vi "Lidar V3.1 RT Main.vi"() -> ()   [LabVIEW 2013]
uses:
  <vilib>/Platform/TimedLoop/XDataNode/timing_clust.ctl
  <vilib>/Platform/TimedLoop/XDataNode/nitl_modes.ctl
  <vilib>/Platform/TimedLoop/XDataNode/wakeup.ctl
  <vilib>/FPGAPlugInAG/PXIe-7962R/niLvFpga_Open_PXIe-7962R.vi
  <vilib>/rvi/interface/common/dynamic/niFpgaDynamicAddResources.vi
  <vilib>/FPGAPlugInAG/Dynamic/niLvFpga_Abort_Dynamic.vi
  <vilib>/FPGAPlugInAG/Dynamic/niLvFpga_Reset_Dynamic.vi
  <vilib>/rvi/interface/common/niFpgaWaitOnOcc.vi
  <vilib>/Utility/error.llb/Error Cluster From Error Code.vi
  <vilib>/FPGAPlugInAG/Dynamic/niLvFpga_Run_Dynamic.vi
  <vilib>/rvi/errors/niLvFpgaAdjustHostInterfaceError.vi
  <vilib>/FPGAPlugInAG/Dynamic/niLvFpga_Close_Dynamic.vi
  <vilib>/rvi/interface/nirviOpenFPGA/nirviOpenFPGA.xnode
  FPGA Bitfiles/GMLIDARV4_FPGATarget3_LIDARV3.1FPGAMai_NnL+G1AkDV4.lvbitx
  <vilib>/rvi/interface/nirviMethod/nirviMethod.xnode
  <vilib>/Platform/TimedLoop/XDataNode/XDataNode.xnode
  <vilib>/rvi/interface/nirviReadWriteControl/nirviReadWriteControl.xnode
  <vilib>/rvi/interface/nirviCloseFPGA/nirviCloseFPGA.xnode
  <vilib>/FPGAPlugInAG/Dynamic/niLvFpga_ReadFifo_Dynamic.vi
  <vilib>/rvi/errors/niLvFpgaMergeErrorWithErrorCode.vi
  <vilib>/ptbypt/NI_PtbyPt.lvlib
  NiFpgaLv.dll
  <vilib>/rvi/interface/Simulation/niFpgaSimulationCallBeginRW.vi
  <vilib>/Platform/TimedLoop/XDataNode/XDNodeRunTimeDep.lvlib
  <vilib>/FPGAPlugInAG/Dynamic/niLvFpga_StopFifo_Dynamic.vi
  <vilib>/FPGAPlugInAG/Dynamic/niLvFpga_ConfigureFifo_Dynamic.vi
  <vilib>/FPGAPlugInAG/Dynamic/niLvFpga_AcquireReadRegionFifo_Dynamic.vi
panel:
  in  "SubstractDark":bool
  out "file path mem":path=path "C:/Users/LIDAR/Desktop/Scans/Debug1.dat"
  in  "SaveDarkFile":bool
  out "Dark Data":dbl[](graph)
  in  "Fill Dark":bool
  in  "SampPerPulse":u16=100 caption="Samples Per Pulse"
  out "Actual Depth 2":u32=4000768
  in  "Mean":bool
  in  "Pilse Wait During Stream":u16=40
  out "SampMem":bool
  in  "# of Frames":u32=1 caption="# of Frames:"
  in  "Frames2File":bool
  in  "Fill VGA":bool
  in  "VGA data":i16[](array[numeric])=[0, 300, 600, 900, 1200, 1500, 1800, 2100, 2400, 2700, 3000, 3300, 3600, 3900, 4200, 4500, 4800, 5100, 5400, 5700, 6000, 6300, 6600, 6900, 7200, 7500, 7800, 8100, 8400, 8700, 9000, 9300, 9600, 9900, 10200, 10500, 10800, 11100, 11400, 11700, 12000, 12300, 12600, 12900, 13200, 13500, 13800, 14100, 14400, 14700, 15000, 15300, 15600, 15900, 16200, 16500, 16800, 17100, 17400, 17700, 18000, 18300, 18600, 18900, 19200, 19500, 19800, 20100, 20400, 20700, 21000, 21300, 21600, 21900, 22200, 22500, 22800, 23100, 23400, 23700, 24000, 24300, 24600, 24900, 25200, 25500, 25800, 26100, 26400, 26700, 27000, 27300, 27600, 27900, 28200, 28500, 28800, 29100, 29400, 29700]
  in  "PulsePerLed":i16=200 caption="Pulses Per Led"
  in  "ScanMode":bool
  in  "FrameStartDisable":bool=TRUE
  out "# of Frames 2":u32
  in  "Frames Stream":bool
  in  "Frames Period":i64=100
  out "Mean Data Timeouts":u16=31333
  out "Actual Depth":u32=4000768
  out "Raw Data Timeouts":u16
  in  "StreamToRawFile":bool
  in  "SingleFrame":bool
  in  "SamplingEnable":bool
  out "Elements":i32=8192
  out "DiskWritesCounter":dbl=6240.0
  out "error out":errorcluster
  in  "Write To File":bool
  in  "file path (use dialog)":path=path "C:/Users/LIDAR/Desktop/Scans/Debug1.dat"
  out "Elements Remaining":u32
  in  "MaxStartSample":u8
  out "Intensity Map":i32[][](graph)=[[4194249, 188752, 224556, 243564, 289464, 295370, 311361, 314977, 331462, 330943, 315425, 258027, 251933, 242647, 177250, 117913], [200096, 226594, 258129, 270777, 343444, 323211, 332534, 349964, 357344, 353930, 351094, 316150, 294820, 265633, 227733, 171654], [232886, 270088, 321175, 342251, 368583, 361813, 383924, 347348, 410423, 416541, 367914, 380971, 350571, 312824, 273514, 214192], [239958, 294260, 316500, 326793, 374683, 379303, 387592, 379517, 393877, 417364, 396781, 427517, 386177, 339906, 293385, 246523], [260822, 288128, 359883, 369758, 370777, 382402, 409421, 424013, 426403, 411324, 377639, 397431, 416573, 383670, 322005, 280464], [293823, 329912, 354981, 353022, 396436, 401968, 405276, 416671, 420226, 421228, 384422, 394623, 423961, 381848, 346743, 317362], [310692, 338310, 379615, 380848, 383413, 440416, 444786, 422715, 400342, 437502, 444652, 443019, 440346, 454579, 408555, 369326], [316804, 342015, 359690, 380257, 428896, 414631, 434872, 421060, 458914, 427260, 480766, 417432, 468249, 416307, 402490, 365401], [303901, 338915, 339851, 378333, 398332, 440528, 418068, 439806, 390220, 406181, 407082, 381751, 436716, 400796, 381358, 367759], [295709, 371852, 371391, 347317, 360777, 398739, 412251, 396109, 380118, 408733, 405717, 414557, 407467, 386729, 398829, 360545], [314919, 350825, 374405, 365676, 393860, 415850, 410229, 441555, 421003, 421694, 496428, 416662, 416732, 423847, 410450, 407682], [328113, 313254, 370853, 381700, 393710, 410688, 382753, 449829, 443229, 458715, 431022, 404412, 413198, 434281, 400200, 423687], [304084, 349902, 347341, 353314, 401704, 422113, 414195, 423142, 395933, 398360, 432970, 390996, 385527, 379727, 377788, 346075], [283824, 313637, 343405, 347712, 394807, 379854, 411027, 383672, 370711, 368886, 401373, 375390, 385415, 371526, 399492, 384905], [260891, 301413, 328721, 319057, 369689, 372537, 399083, 380860, 364897, 382376, 427845, 447504, 378799, 362669, 372146, 366827], [260673, 275664, 297429, 325884, 386054, 389853, 378447, 387074, 385946, 363162, 422310, 380432, 373896, 375205, 367301, 363228], [275808, 284523, 294765, 333943, 308894, 378299, 378336, 357836, 389531, 381008, 372799, 357010, 370219, 350399, 328994, 324885], [232169, 242832, 279229, 299502, 307673, 352062, 346701, 334907, 340086, 344861, 384207, 371964, 357009, 350037, 361186, 312514], [217595, 247026, 267875, 295673, 319858, 333157, 327430, 316329, 320075, 324786, 310662, 357832, 315871, 368283, 331984, 254258], [210648, 254981, 278468, 289551, 280066, 318278, 342140, 319921, 320714, 335552, 365830, 364916, 332478, 350151, 315016, 244036]]
  in  "ActiveLedIndex":u16=144
  in  "LedScanDebEn":bool
  in  "LaserPower 1":bool=TRUE
  in  "LaserPower 0":bool=TRUE
  out "Range Map":u32[][](graph)=[[0, 62009, 61985, 61985, 62033, 61985, 61985, 62033, 62033, 62033, 62057, 62165, 62117, 62033, 62117, 62357], [61865, 61925, 62021, 61985, 62057, 62045, 62081, 62129, 62093, 62093, 62069, 62057, 62069, 62069, 62021, 61985], [62201, 62285, 62261, 62321, 62297, 62357, 62357, 62393, 62189, 62213, 62225, 62189, 62201, 62261, 62321, 62357], [62381, 62357, 62405, 62357, 62333, 62381, 62393, 62429, 62297, 62297, 62285, 62297, 62285, 62273, 62297, 62357], [61841, 61901, 61997, 61973, 61973, 62045, 62009, 62033, 62081, 62081, 62117, 62069, 62105, 61997, 62033, 61961], [61973, 61961, 61973, 61961, 61997, 62033, 62033, 62057, 62117, 62081, 62141, 62141, 62117, 62069, 62009, 61973], [62201, 62249, 62237, 62249, 62285, 62285, 62249, 62297, 62201, 62189, 62177, 62225, 62177, 62117, 62069, 62105], [62261, 62357, 62357, 62357, 62297, 62381, 62357, 62357, 62189, 62273, 62225, 62297, 62261, 62273, 62201, 62141], [61709, 61745, 61757, 61733, 61733, 61745, 61769, 61793, 61889, 61901, 61901, 61937, 61913, 61889, 61877, 61841], [61721, 61733, 61745, 61733, 61745, 61757, 61745, 61781, 61901, 61877, 61913, 61925, 61937, 61865, 61865, 61841], [62009, 62009, 62033, 62021, 61997, 62009, 62021, 62021, 61949, 61973, 61949, 61997, 62009, 61961, 61973, 61937], [61853, 61889, 61889, 61853, 61877, 61877, 61901, 61865, 61757, 61793, 61805, 61841, 61841, 61793, 61793, 61781], [61541, 61541, 61565, 61541, 61541, 61541, 61541, 61565, 61589, 61613, 61625, 61637, 61637, 61601, 61613, 61625], [61733, 61733, 61733, 61721, 61721, 61733, 61733, 61721, 61781, 61793, 61829, 61817, 61829, 61817, 61817, 61829], [61769, 61769, 61769, 61769, 61745, 61769, 61793, 61781, 61709, 61721, 61697, 61733, 61733, 61733, 61709, 61709], [61769, 61781, 61805, 61769, 61745, 61781, 61793, 61793, 61673, 61721, 61709, 61709, 61721, 61697, 61709, 61685], [61541, 61541, 61541, 61517, 61529, 61565, 61565, 61529, 61577, 61577, 61589, 61589, 61601, 61565, 61577, 61589], [61529, 61505, 61529, 61505, 61541, 61529, 61529, 61529, 61589, 61589, 61637, 61625, 61637, 61613, 61625, 61601], [61745, 61745, 61745, 61733, 61721, 61733, 61745, 61745, 61673, 61685, 61685, 61697, 61709, 61685, 61673, 61721], [61637, 61601, 61625, 61601, 61613, 61625, 61625, 61625, 61553, 61553, 61553, 61577, 61589, 61553, 61553, 31574]]
  in  "PulseEndClock":u8=4
  in  "PulseWaitClck":u16
  in  "Freq [Mhz]":dbl=125000000.0 format="%#_6p"
  out "standard deviation":dbl format="%0.5f"
  out "Distance":dbl format="%#.4f"
  in  "stop":bool=TRUE
  # "Auto Actions"
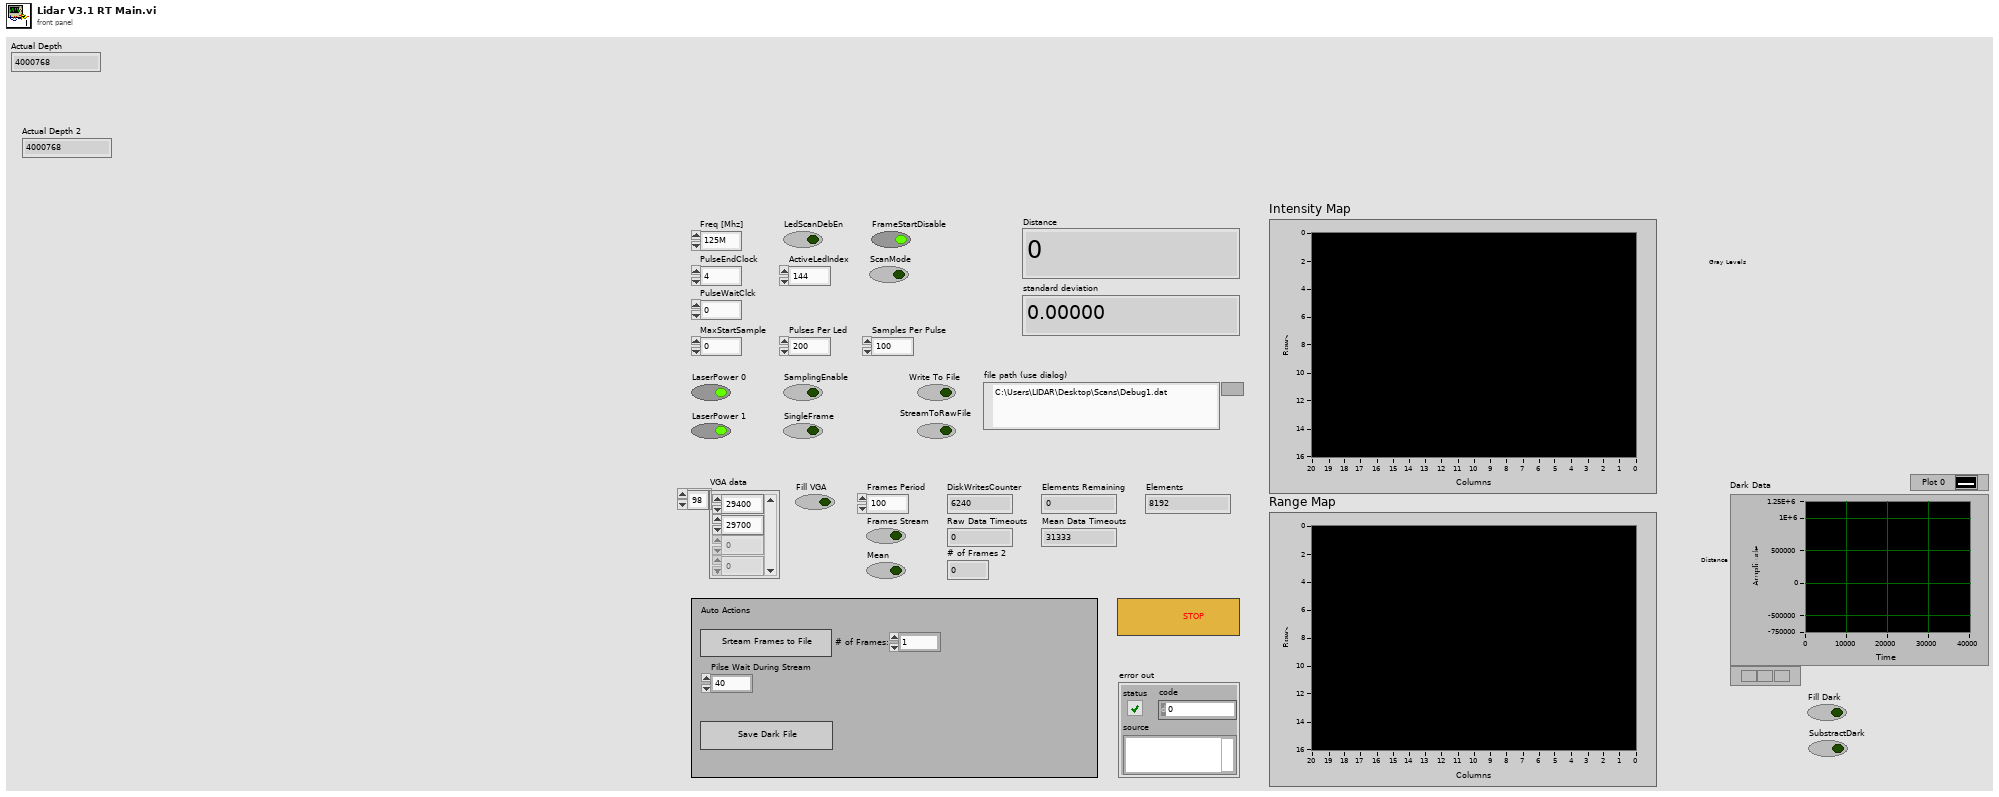
[diagram p1: front panel]
types:
  T1 = typedef "XDNodeRunTimeDep.lvlib/timing_clust.ctl" = cluster{"Expected End [f-1]":u64, "Actual End [f-1]":u64, "Finished Late? [f-1]":bool, "Expected End [i-1]":u64, "Actual End [i-1]":u64, "Finished Late? [i-1]":bool, "Expected Start [i]":u64, "Actual Start [i]":u64, "Expected Start [f]":u64, "Actual Start [f]":u64, "Source Name":string, "Structure Name":string, "Period":i64, "Deadline":i64, "Offset":i64, "Start":i64, "Priority":i32, "Timeout":i32, "Mode":T2, "Wakeup Reason":T3, "Error":errorcluster, "Source Type":string, "Secondary Source Type":string, "Global End Time":u64, "Global Start Time":u64, "Frame Duration":u64, "Iteration Duration":u64, "Assigned CPU":i32, "I/O Scan Engine Mode":u32}
  T2 = typedef "XDNodeRunTimeDep.lvlib/nitl_modes.ctl" = enum32{"No Change", "Process missed periods, maintain original phase", "Discard missed periods, maintain original phase", "Process missed periods, ignore original phase", "Discard missed periods, ignore original phase"}
  T3 = typedef "XDNodeRunTimeDep.lvlib/wakeup.ctl" = enum32{"Normal", "Aborted", "Asynchronous wakeup", "Timing source error", "Timed loop error", "Timeout"}
  T4 = enum16{"open", "replace", "create", "open or create", "replace or create", "replace or create with confirmation"}
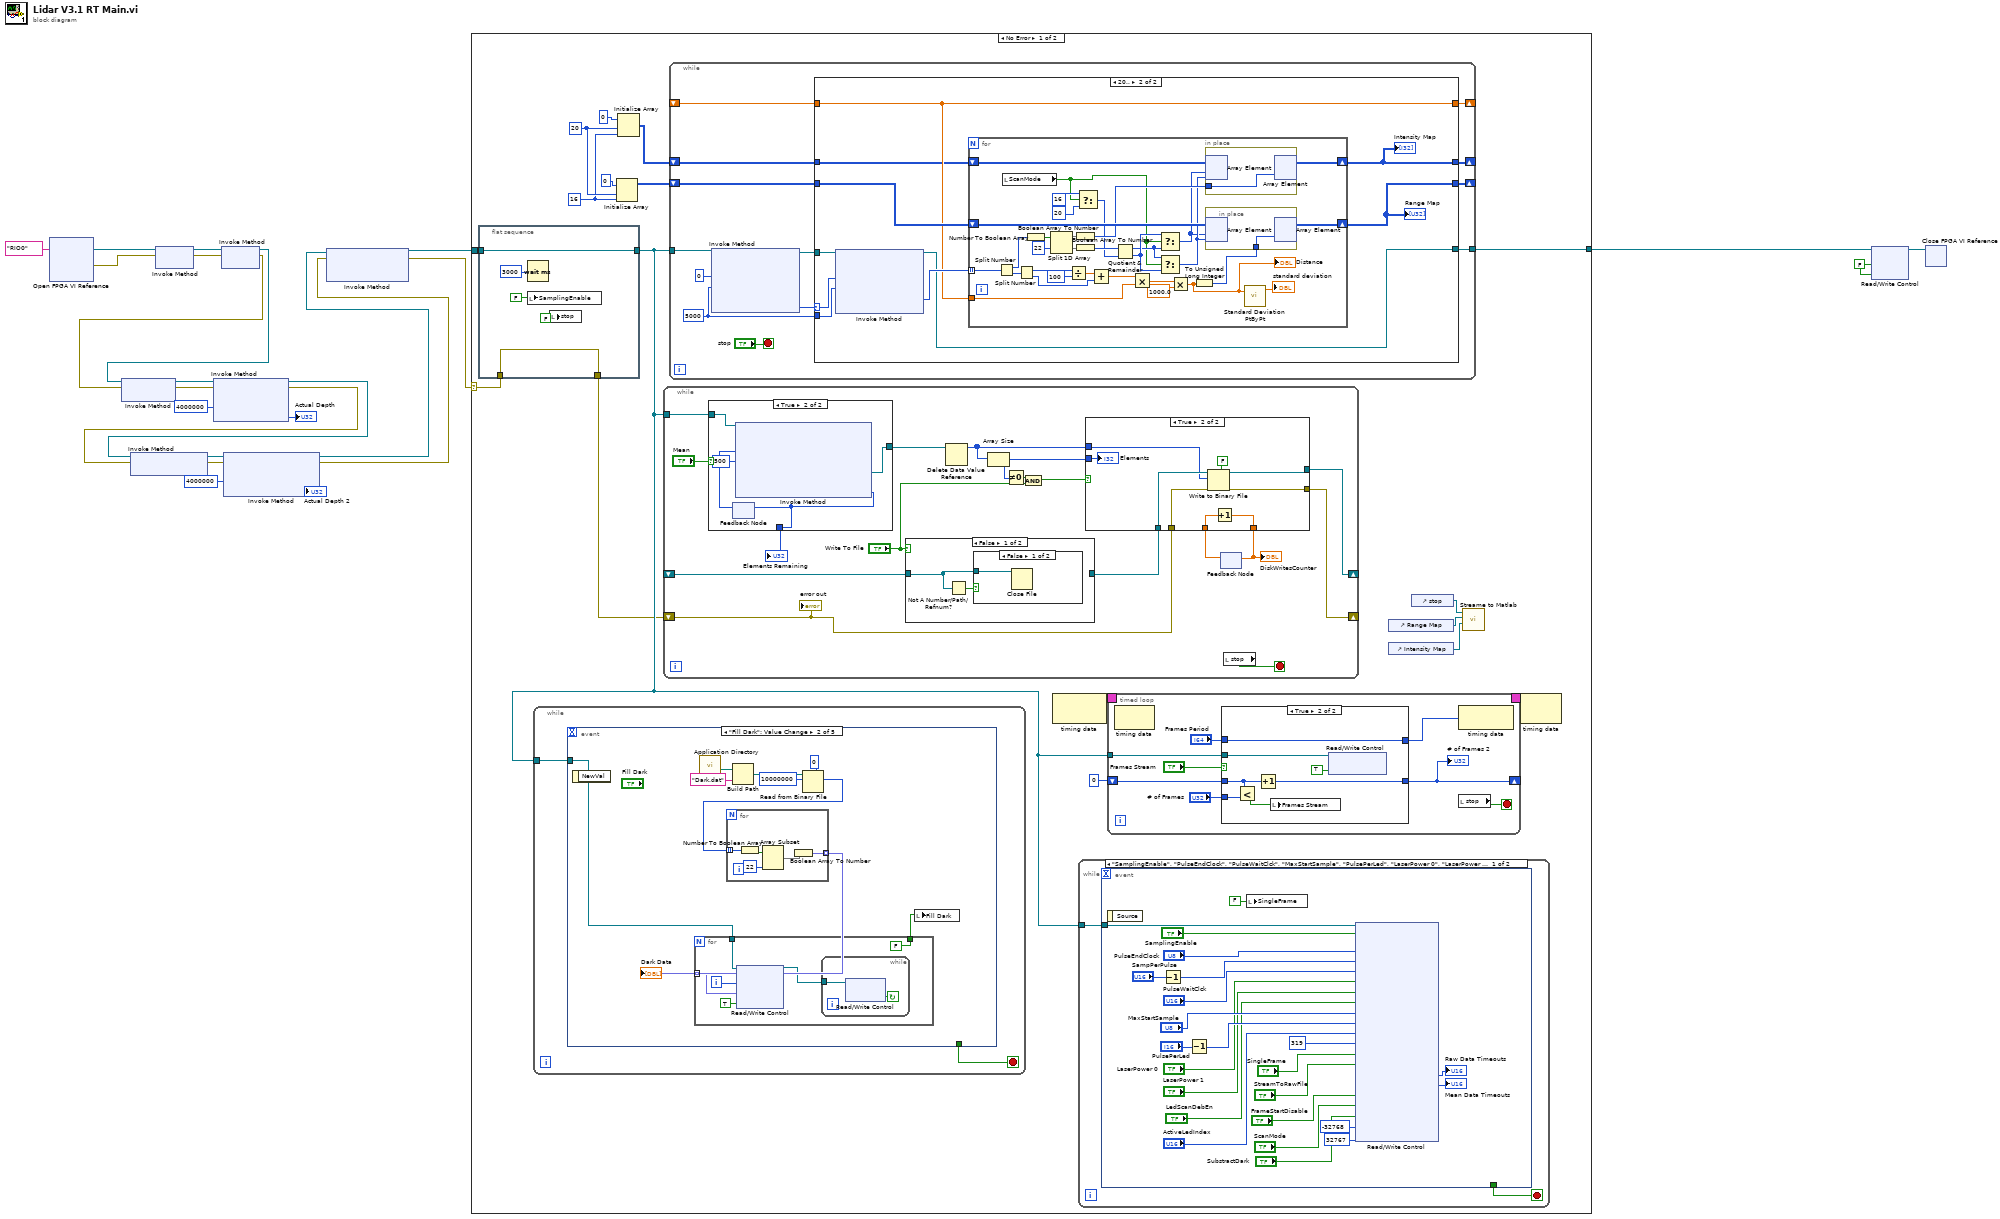
[diagram p0: block diagram]
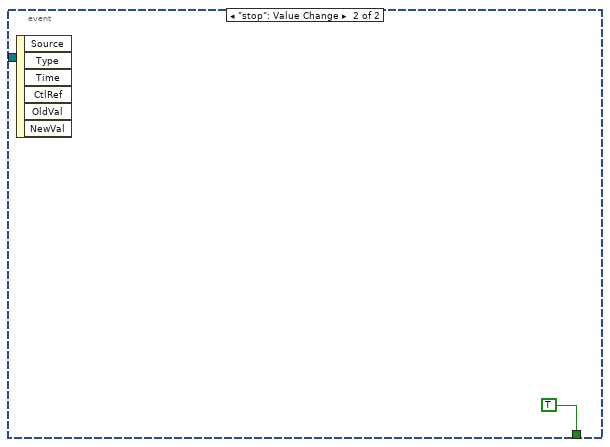
[diagram p2: hidden frame]
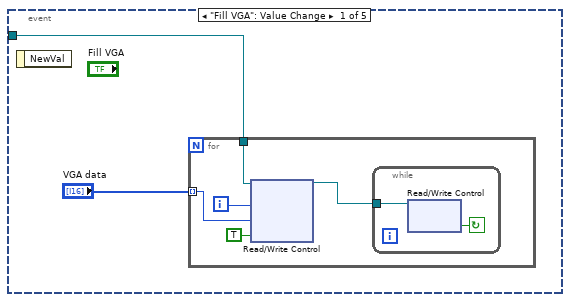
[diagram p3: hidden frame]
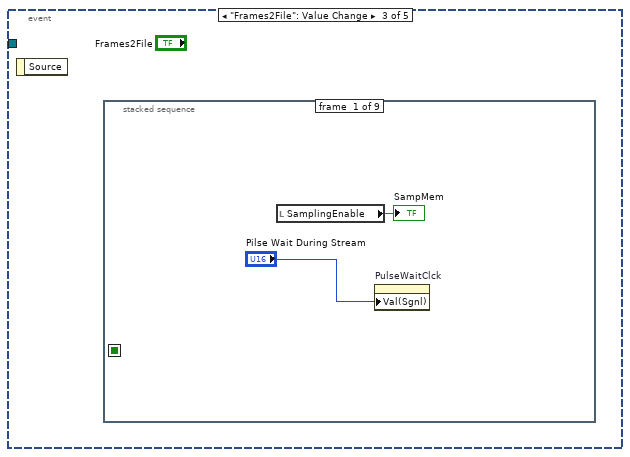
[diagram p4: hidden frame]
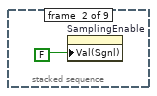
[diagram p5: hidden frame]
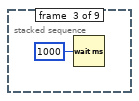
[diagram p6: hidden frame]
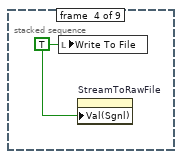
[diagram p7: hidden frame]
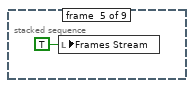
[diagram p8: hidden frame]
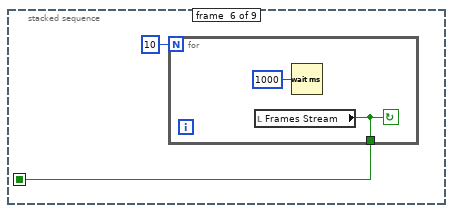
[diagram p9: hidden frame]
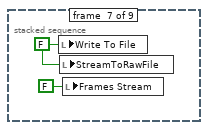
[diagram p10: hidden frame]
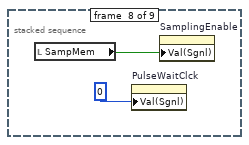
[diagram p11: hidden frame]
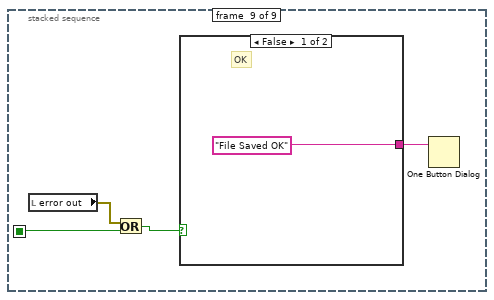
[diagram p12: hidden frame]
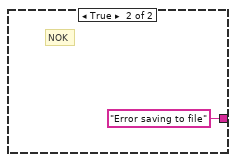
[diagram p13: hidden frame]
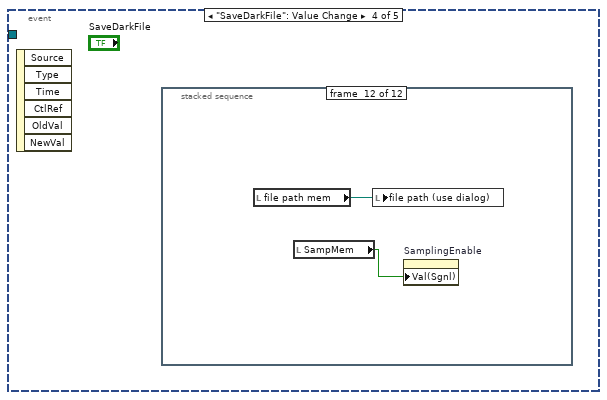
[diagram p14: hidden frame]
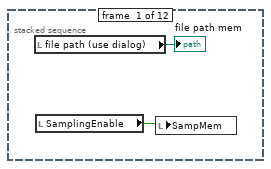
[diagram p15: hidden frame]
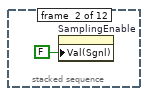
[diagram p16: hidden frame]
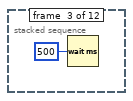
[diagram p17: hidden frame]
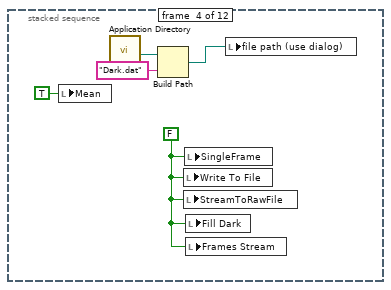
[diagram p18: hidden frame]
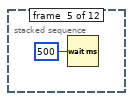
[diagram p19: hidden frame]
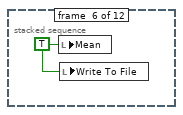
[diagram p20: hidden frame]
diagram:
  w14 = FALSE ("PFI2")
  n1 = xnode "Open FPGA VI Reference"("resource name"=tag "RIO0") -> ("FPGA VI Reference Out"=w22:refnum<k20>, "error out"=w20:errorcluster)  [unwired: 1 in]
  n2 = xnode "Invoke Method"("FPGA VI Reference In"=w22, "error in"=w20) -> ("FPGA VI Reference Out"=w21:refnum<k20>, "error out"=w19:errorcluster)
  n3 = xnode "Invoke Method"("FPGA VI Reference In"=w21, "error in"=w19) -> ("FPGA VI Reference Out"=w6:refnum<k20>, "error out"=w5:errorcluster)
  n4 = xnode "Invoke Method"("FPGA VI Reference In"=w6, "error in"=w5) -> ("FPGA VI Reference Out"=w17:refnum<k20>, "error out"=w18:errorcluster)
  n5 = xnode "Invoke Method"("FPGA VI Reference In"=w17, "error in"=w18, "Requested Depth"=u32 4000000) -> ("FPGA VI Reference Out"=w8:refnum<k20>, "error out"=w7:errorcluster, "Actual Depth"=→"Actual Depth":u32)
  n6 = xnode "Invoke Method"("FPGA VI Reference In"=w8, "error in"=w7) -> ("FPGA VI Reference Out"=w10:refnum<k20>, "error out"=w9:errorcluster)
  n7 = xnode "Invoke Method"("FPGA VI Reference In"=w10, "error in"=w9, "Requested Depth"=u32 4000000) -> ("FPGA VI Reference Out"=w4:refnum<k20>, "error out"=w2:errorcluster, "Actual Depth"=→"Actual Depth 2":u32)
  n8 = xnode "Invoke Method"("FPGA VI Reference In"=w4, "error in"=w2) -> ("FPGA VI Reference Out"=w3:refnum<k20>, "error out"=w1:errorcluster)  [unwired: 1 in]
  n9 = case shown="No Error" w1 {
    selector: w1 -> [w29 w285]
    tunnel: [w39 w286] -> w23
    tunnel: w3 -> [w31 w286]
    frame No Error {
      w32 = 16 ("dimension size")
      w36 = 20 ("dimension size")
      n10 = flat-sequence {
        tunnel: [w145] -> w30
        tunnel: w31 -> [w145]
        tunnel: w29 -> [w141]
        tunnel: [w141] -> w28
        frame #0 {
          n11 = Wait (ms)(milliseconds to wait=u32 3000) -> ()  [unwired: 1 out]
          n12 = local write "SamplingEnable"(FALSE ("SamplingEnable")) -> ()
          n13 = local write "stop"(FALSE ("stop")) -> ()
        }
      }
      n14 = while {
        tunnel: w30 -> [w70]
        stop <- w69 stop-if-true
        n15 = event shown="[1] \"Fill Dark\": Value Change" {
          selector: _ -> [_ _ _ _ _]
          dyn-events: _ -> [_ _ _ _ _]
          timeout: _ -> [_ _ _ _ _]
          tunnel: w70 -> [w71 w83 _ _ _]
          tunnel: [_ _ _ _ TRUE] -> w69
          event "Fill VGA": Value Change {
            n16 = event-data() -> ()  [unwired: 1 in, 1 out]
            n17 = for {
              tunnel: w71 -> [w77]
              tunnel: "VGA data" -> [w76] mode=indexing
              i -> [w75]
              n18 = xnode "Read/Write Control"("FPGA VI Reference In"=w77, "VgaAdd"=w75, "VgaData"=w76, "FillVga"=TRUE) -> ("FPGA VI Reference Out"=w74:refnum<k20>)  [unwired: 1 in, 1 out]
              n19 = while {
                tunnel: w74 -> [w79]
                stop <- w78 continue-if-true
                n20 = xnode "Read/Write Control"("FPGA VI Reference In"=w79) -> ("FillVga"=w78:bool)  [unwired: 1 in, 2 out]
              }
            }
          }
          event "Fill Dark": Value Change {
            n21 = event-data() -> ()  [unwired: 1 in, 1 out]
            n22 = call <vilib>:"Application Directory.vi"() -> ("Application Directory"=w88:path)
            n23 = Build Path(base path=w88, name or relative path="Dark.dat") -> (appended path=w84:path)
            n24 = Read from Binary File(5:u32 0, 10:10000000 ("count (1)"), 11:w84) -> (2:w81:u32[])  [unwired: 3 in, 3 out]
            n25 = for {
              tunnel: w81 -> [w93] mode=indexing
              tunnel: [w89] -> w80 mode=indexing
              n26 = Number To Boolean Array(number=w93) -> (Boolean array=w92:bool[])
              n27 = Array Subset(array=w92, length=22) -> (w90:bool[])  [unwired: 1 in]
              n28 = Boolean Array To Number(Boolean array=w90) -> (number=w89:fxp<+/-,22,22>)
            }
            "Dark Data" <- w80
            n29 = for {
              tunnel: w83 -> [w99]
              tunnel: w80 -> [w94] mode=indexing
              tunnel: [FALSE] -> w82
              i -> [w98]
              n30 = xnode "Read/Write Control"("FPGA VI Reference In"=w99, "DarkAdd"=w98, "DarkData"=w94, "FillDark"=TRUE ("FillVga")) -> ("FPGA VI Reference Out"=w97:refnum<k20>)  [unwired: 1 in, 1 out]
              n31 = while {
                tunnel: w97 -> [w101]
                stop <- w100 continue-if-true
                n32 = xnode "Read/Write Control"("FPGA VI Reference In"=w101) -> ("FillDark"=w100:bool)  [unwired: 1 in, 2 out]
              }
            }
            n33 = local write "Fill Dark"(w82) -> ()
          }
          event "Frames2File": Value Change {
            n34 = event-data() -> ()  [unwired: 1 in, 1 out]
            n35 = stacked-sequence {
              seq-local: [_ _ _ _ _ w108 _ _ _] -> [_ _ _ _ _ _ _ _ w119]
              frame #0 {
                n36 = local read "SamplingEnable"() -> (→"SampMem":bool)
                n37 = property on="PulseWaitClck" class="DigNum (strict)"("Val(Sgnl)"="Pilse Wait During Stream") -> ()  [unwired: 2 in, 2 out]
              }
              frame #1 {
                n38 = property on="SamplingEnable" class="Bool (strict)"("Val(Sgnl)"=FALSE ("SamplingEnable")) -> ()  [unwired: 2 in, 2 out]
              }
              frame #2 {
                n39 = Wait (ms)(milliseconds to wait=u32 1000) -> ()  [unwired: 1 out]
              }
              frame #3 {
                w106 = TRUE ("Write To File")
                n40 = local write "Write To File"(w106) -> ()
                n41 = property on="StreamToRawFile" class="Bool (strict)"("Val(Sgnl)"=w106) -> ()  [unwired: 2 in, 2 out]
              }
              frame #4 {
                n42 = local write "Frames Stream"(TRUE ("Frames Stream")) -> ()
              }
              frame #5 {
                n43 = for {
                  N: 10 -> [_]
                  tunnel: [w110] -> w108
                  stop <- w110 continue-if-true
                  n44 = local read "Frames Stream"() -> (w110:bool)
                  n45 = Wait (ms)(milliseconds to wait=u32 1000) -> ()  [unwired: 1 out]
                }
              }
              frame #6 {
                w112 = FALSE ("Write To File")
                n46 = local write "Write To File"(w112) -> ()
                n47 = local write "StreamToRawFile"(w112) -> ()
                n48 = local write "Frames Stream"(FALSE ("Frames Stream")) -> ()
              }
              frame #7 {
                n49 = local read "SampMem"() -> (w115:bool)
                n50 = property on="PulseWaitClck" class="DigNum (strict)"("Val(Sgnl)"=u16 0 ("PulseWaitClck")) -> ()  [unwired: 2 in, 2 out]
                n51 = property on="SamplingEnable" class="Bool (strict)"("Val(Sgnl)"=w115) -> ()  [unwired: 2 in, 2 out]
              }
              frame #8 {
                n52 = local read "error out"() -> (w116:errorcluster)
                n53 = Or(x=w116, y=w119) -> (x .or. y?=w117:bool)
                n54 = case shown="False" w117 {
                  tunnel: ["File Saved OK" ("message") "Error saving to file" ("message")] -> w118
                  frame False {
                    # "OK"
                  }
                  frame True {
                    # "NOK"
                  }
                }
                n55 = One Button Dialog(message=w118) -> ()  [unwired: 1 in, 1 out]
              }
            }
          }
          event "SaveDarkFile": Value Change {
            n56 = event-data() -> ()  [unwired: 1 in, 6 out]
            n57 = stacked-sequence {
              frame #0 {
                n58 = local read "file path (use dialog)"() -> (→"file path mem":path)
                n59 = local read "SamplingEnable"() -> (w123:bool)
                n60 = local write "SampMem"(w123) -> ()
              }
              frame #1 {
                n61 = property on="SamplingEnable" class="Bool (strict)"("Val(Sgnl)"=FALSE ("Value (Signaling)")) -> ()  [unwired: 2 in, 2 out]
              }
              frame #2 {
                n62 = Wait (ms)(milliseconds to wait=u32 500) -> ()  [unwired: 1 out]
              }
              frame #3 {
                w126 = FALSE ("SamplingEnable")
                n63 = local write "Mean"(TRUE ("Mean")) -> ()
                n64 = call <vilib>:"Application Directory.vi"() -> ("Application Directory"=w130:path)
                n65 = Build Path(base path=w130, name or relative path="Dark.dat") -> (appended path=w128:path)
                n66 = local write "Write To File"(w126) -> ()
                n67 = local write "StreamToRawFile"(w126) -> ()
                n68 = local write "SingleFrame"(w126) -> ()
                n69 = local write "Fill Dark"(w126) -> ()
                n70 = local write "Frames Stream"(w126) -> ()
                n71 = local write "file path (use dialog)"(w128) -> ()
              }
              frame #4 {
                n72 = Wait (ms)(milliseconds to wait=u32 500) -> ()  [unwired: 1 out]
              }
              frame #5 {
                w132 = TRUE ("Mean")
                n73 = local write "Mean"(w132) -> ()
                n74 = local write "Write To File"(w132) -> ()
              }
              frame #6 {
                n75 = Wait (ms)(milliseconds to wait=u32 500) -> ()  [unwired: 1 out]
              }
              frame #7 {
                n76 = property on="SingleFrame" class="Bool (strict)"("Val(Sgnl)"=TRUE ("SingleFrame")) -> ()  [unwired: 2 in, 2 out]
              }
              frame #8 {
                n77 = Wait (ms)(milliseconds to wait=u32 1000) -> ()  [unwired: 1 out]
              }
              frame #9 {
                w136 = FALSE ("SamplingEnable")
                n78 = local write "Write To File"(w136) -> ()
                n79 = local write "StreamToRawFile"(w136) -> ()
                n80 = local write "SingleFrame"(w136) -> ()
                n81 = local write "Fill Dark"(w136) -> ()
                n82 = local write "Frames Stream"(w136) -> ()
                n83 = local write "SamplingEnable"(w136) -> ()
                n84 = local write "Mean"(w136) -> ()
              }
              frame #10 {
                n85 = Wait (ms)(milliseconds to wait=u32 1000) -> ()  [unwired: 1 out]
              }
              frame #11 {
                n86 = local read "file path mem"() -> (w139:path)
                n87 = local read "SampMem"() -> (w138:bool)
                n88 = local write "file path (use dialog)"(w139) -> ()
                n89 = property on="SamplingEnable" class="Bool (strict)"("Val(Sgnl)"=w138) -> ()  [unwired: 2 in, 2 out]
              }
            }
          }
          event "stop": Value Change {
            n90 = event-data() -> ()  [unwired: 1 in, 6 out]
          }
        }
      }
      n91 = Initialize Array(u32 0 ("element"), w36, w32) -> (w37:u32[][])
      n92 = Initialize Array(0 ("element"), w36, w32) -> (w34:i32[][])
      n93 = while {
        tunnel: w30 -> [w184]
        shift-right: [w183] -> _
        shift-left: _ -> [w176]
        shift-right: [w182] -> _
        shift-left: w28 -> [w181]
        stop <- w170 stop-if-true
        n94 = case shown="True" "Mean" {
          tunnel: w184 -> [w189 w194]
          tunnel: [w188 w193] -> w178
          tunnel: [w186 w190] -> w169
          frame False {
            n95 = feedback #1() -> (w185:u32)  [unwired: 1 in]
            n96 = xnode "Invoke Method"("FPGA VI Reference In"=w189, "Number of Elements"=w185, "Timeout (ms)"=500) -> ("Read Region Reference"=w188:refnum<data-value>, "Elements Remaining"=w186:u32)  [unwired: 1 in, 3 out]
            n97 = feedback-in #1(w186) -> ()
          }
          frame True {
            n98 = feedback #2() -> (w191:u32)  [unwired: 1 in]
            n99 = xnode "Invoke Method"("FPGA VI Reference In"=w194, "Number of Elements"=w191, "Timeout (ms)"=500) -> ("Read Region Reference"=w193:refnum<data-value>, "Elements Remaining"=w190:u32)  [unwired: 1 in, 3 out]
            n100 = feedback-in #2(w190) -> ()
          }
        }
        "Elements Remaining" <- w169
        n101 = case shown="False" "Write To File" {
          tunnel: w176 -> [w195 w198]
          tunnel: [_ w200] -> w175
          frame False {
            n102 = Not A Number/Path/Refnum?(number/path/refnum=w195) -> (NaN/Path/Refnum?=w196:bool)
            n103 = case shown="False" w196 {
              tunnel: w195 -> [w197 _]
              frame False {
                n104 = Close File(refnum=w197) -> ()  [unwired: 1 in, 2 out]
              }
              frame True {
              }
            }
          }
          frame True {
            n105 = Not A Number/Path/Refnum?(number/path/refnum=w198) -> (NaN/Path/Refnum?=w199:bool)
            n106 = case shown="True" w199 {
              tunnel: [w201 w202] -> w200
              tunnel: w198 -> [w201 _]
              frame False {
              }
              frame True {
                n107 = Open/Create/Replace File(file path (use dialog)="file path (use dialog)", operation (0:open)=T4."replace or create") -> (refnum out=w202:refnum<file>)  [unwired: 4 in, 2 out]
              }
            }
          }
        }
        n108 = Delete Data Value Reference(data value reference=w178) -> (data value=w173:u32[])  [unwired: 1 in, 1 out]
        n109 = Array Size(array=w173) -> (size(s)=w172:i32)
        n110 = Not Equal To 0?(x=w172) -> (x != 0?=w171:bool)
        n111 = And(x=w171, y="Write To File") -> (x .and. y?=w177:bool)
        n112 = feedback #3() -> (w179:dbl)  [unwired: 1 in]
        n113 = case shown="True" w177 {
          tunnel: [w205 w215] -> w183
          tunnel: w181 -> [w207 w210]
          tunnel: [w207 w214] -> w182
          tunnel: [w206 w212] -> w180
          tunnel: w179 -> [w206 w213]
          tunnel: w173 -> [_ w209]
          tunnel: w175 -> [w205 w211]
          tunnel: w172 -> [_ w208]
          frame False {
          }
          frame True {
            n114 = Write to Binary File(file (use dialog)=w211, data=w209, error in=w210, 5:FALSE ("prepend array or string size? (T)")) -> (refnum out=w215:refnum<file>, error out=w214:errorcluster)  [unwired: 2 in, 1 out]
            n115 = Increment(x=w213) -> (x+1=w212:dbl)
            "Elements" <- w208
          }
        }
        "DiskWritesCounter" <- w180
        n116 = feedback-in #3(w180) -> ()
        n117 = local read "stop"() -> (w170:bool)
        "error out" <- w181
      }
      n118 = while {
        tunnel: w30 -> [w229]
        tunnel: [w224] -> w39
        shift-right: [w222] -> _
        shift-left: _ -> [w221]
        shift-right: [w219] -> _
        shift-left: w37 -> [w220]
        shift-right: [w217] -> _
        shift-left: w34 -> [w218]
        stop <- "stop" stop-if-true
        w226 = 5000 ("Timeout (ms)")
        n119 = xnode "Invoke Method"("FPGA VI Reference In"=w229, "Number of Elements"=u32 0, "Timeout (ms)"=w226) -> ("FPGA VI Reference Out"=w227:refnum<k20>, "Elements Remaining"=w223:u32)  [unwired: 1 in, 2 out]
        n120 = case shown="20.." w223 {
          selector: w223 -> [_ w243]
          tunnel: w227 -> [w240 w250]
          tunnel: w226 -> [_ w249]
          tunnel: [w240 w247] -> w224
          tunnel: [w232 w245] -> w222
          tunnel: w221 -> [_ w245]
          tunnel: w220 -> [w231 w246]
          tunnel: [w231 w242] -> w219
          tunnel: w218 -> [w230 w244]
          tunnel: [w230 w241] -> w217
          frame Default {
            n121 = Reciprocal(x="Freq [Mhz]") -> (1/x=w239:dbl)
            n122 = Multiply(x=w239, y=dbl[unit] 299792458.0) -> (x*y=w236:dbl[unit])
            n123 = Multiply(x=w236, y=dbl[unit] 0.5) -> (x*y=w233:dbl[unit])
            n124 = Type Cast(type=0.0 ("y"), x=w233) -> (*(type *) &x=w232:dbl)
          }
          frame 20.. {
            n125 = xnode "Invoke Method"("FPGA VI Reference In"=w250, "Number of Elements"=w243, "Timeout (ms)"=w249) -> ("FPGA VI Reference Out"=w247:refnum<k20>, "Data"=w248:u64[])  [unwired: 1 in, 2 out]
            n126 = for {
              tunnel: w248 -> [w282] mode=indexing
              shift-right: [w278] -> w242
              shift-left: w246 -> [w279]
              tunnel: w245 -> [w277]
              shift-right: [w274] -> w241
              shift-left: w244 -> [w275]
              n127 = Split Number(x=w282) -> (hi(x)=w280:u32, lo(x)=w281:u32)
              n128 = local read "ScanMode"() -> (w251:bool)
              n129 = Split Number(x=w281) -> (hi(x)=w276:u16, lo(x)=w273:u16)
              n130 = Number To Boolean Array(number=w280) -> (Boolean array=w272:bool[])
              n131 = Split 1D Array(array=w272, index=22) -> (first subarray=w262:bool[], second subarray=w270:bool[])
              n132 = Divide(x=w276, y=u16 100) -> (x/y=w267:dbl)
              n133 = Boolean Array To Number(Boolean array=w262) -> (number=w261:i32)
              n134 = Boolean Array To Number(Boolean array=w270) -> (number=w269:u32)
              n135 = Select(t=u32 16 ("y"), s=w251, f=u32 20 ("y")) -> (s? t:f=w257:u32)
              n136 = Add(x=w267, y=w273) -> (x+y=w268:dbl)
              n137 = Quotient & Remainder(x=w269, y=w257) -> (x-y*floor(x/y)=w252:u32, floor(x/y)=w253:u32)
              n138 = Multiply(x=w268, y=w277) -> (x*y=w264:dbl)
              n139 = Select(t=w253, s=w251, f=w252) -> (s? t:f=w254:u32)
              n140 = Select(t=w252, s=w251, f=w253) -> (s? t:f=w255:u32)
              n141 = Multiply(x=w264, y=1000.0) -> (x*y=w260:dbl)
              "Distance" <- w260
              n142 = To Unsigned Long Integer(number=w260) -> (unsigned 32bit integer=w259:u32)
              n143 = in-place {
                in-place-border: w261 -> [w283]
                n144 = in-place-array #4(w275, w254, w255) -> ()  [unwired: 1 out]
                n145 = in-place-array #4(w283) -> (w274:i32[][])  [unwired: 2 out]
              }
              n146 = in-place {
                in-place-border: w259 -> [w284]
                n147 = in-place-array #5(w279, w254, w255) -> ()  [unwired: 1 out]
                n148 = in-place-array #5(w284) -> (w278:u32[][])  [unwired: 2 out]
              }
              n149 = call <vilib>:"Standard Deviation PtByPt.vi"("x"=w260) -> ("standard deviation"=→"standard deviation":dbl)  [unwired: 2 in, 2 out]
            }
            "Range Map" <- w242
            "Intensity Map" <- w241
          }
        }
      }
      n150 = node-c288() -> (w41:T1)  [unwired: 1 in]
      n151 = while {
        tunnel: w30 -> [w42]
        stop <- w43 stop-if-true
        n152 = event shown="[0] \"SamplingEnable\", \"PulseEndClock\", \"PulseWaitClck\", \"MaxStartSample\", \"PulsePerLed\", \"LaserPower 0\", \"LaserPower 1\", \"LedScanDebEn\", \"ActiveLedIndex\", \"SingleFrame\", \"StreamToRawFile\", \"FrameStartDisable\", \"ScanMode\", \"SubstractDark\": Value Change" {
          selector: _ -> [_ _]
          dyn-events: _ -> [_ _]
          timeout: _ -> [_ _]
          tunnel: [_ TRUE] -> w43
          tunnel: w42 -> [w50 _]
          event "SamplingEnable", "PulseEndClock", "PulseWaitClck", "MaxStartSample", "PulsePerLed", "LaserPower 0", "LaserPower 1", "LedScanDebEn", "ActiveLedIndex", "SingleFrame", "StreamToRawFile", "FrameStartDisable", "ScanMode", "SubstractDark": Value Change {
            n153 = event-data() -> ()  [unwired: 1 in, 1 out]
            n154 = Decrement(x="SampPerPulse") -> (x-1=w48:u16)
            n155 = Decrement(x="PulsePerLed") -> (x-1=w67:i16)
            n156 = local write "SingleFrame"(FALSE ("SingleFrame")) -> ()
            n157 = xnode "Read/Write Control"("FPGA VI Reference In"=w50, "SamplingEnable"="SamplingEnable", "PulseEndClck"="PulseEndClock", "SampPerPulse"=w48, "PulseWaitClck"="PulseWaitClck", "PFI2"="LaserPower 0", "PFI3"="LaserPower 1", "LedScanDebEn"="LedScanDebEn", "MaxStartSample"="MaxStartSample", "PulsePerLed"=w67, "ActiveLedIndexDeb"="ActiveLedIndex", "NoOfLeds"=u16 319, "SingleFrame"="SingleFrame", "StreamToDMA"="StreamToRawFile", "FrameStartDisable"="FrameStartDisable", "ScanMode"="ScanMode", "SubstractDark"="SubstractDark", "OutOFFValue"=i16 -32768, "OutONValue"=i16 32767) -> ("Timeouts"=→"Raw Data Timeouts":u16, "MeanTimeouts"=→"Mean Data Timeouts":u16)  [unwired: 1 in, 2 out]
          }
          event "stop": Value Change {
            n158 = event-data() -> ()  [unwired: 1 in, 6 out]
          }
        }
      }
      n159 = timed-loop {
        timing: w41 -> [_]
        timing-out: [_] -> w40
        tunnel: w30 -> [w153]
        shift-right: [w148] -> _
        shift-left: u32 0 ("# of Frames") -> [w149]
        stop <- w150 stop-if-true
        n160 = node-c288() -> ()  [unwired: 1 in, 1 out]
        n161 = case shown="True" "Frames Stream" {
          tunnel: w153 -> [_ w161]
          tunnel: [i64 1000 ("Frames Period") w160] -> w151
          tunnel: "Frames Period" -> [_ w160]
          tunnel: w149 -> [_ w156]
          tunnel: [_ w159] -> w148
          tunnel: "# of Frames" -> [_ w157]
          frame False {
          }
          frame True {
            n162 = Less?(x=w156, y=w157) -> (x < y?=w155:bool)
            n163 = Increment(x=w156) -> (x+1=w159:u32)
            n164 = local write "Frames Stream"(w155) -> ()
            n165 = xnode "Read/Write Control"("FPGA VI Reference In"=w161, "SingleFrame"=TRUE) -> ()  [unwired: 1 in, 2 out]
          }
        }
        "# of Frames 2" <- w148
        n166 = node-c288(w151) -> ()  [unwired: 1 out]
        n167 = local read "stop"() -> (w150:bool)
      }
      n168 = control-ref of="Range Map"() -> (w26:refnum<vi>)
      n169 = control-ref of="Intensity Map"() -> (w25:refnum<vi>)
      n170 = control-ref of="stop"() -> (w27:refnum<vi>)
      n171 = call "Streame to Matlab.vi"("Intensity"=w25, "range"=w26, "StopRef"=w27) -> ()  [unwired: 9 in]
      n172 = node-c288(w40) -> ()  [unwired: 1 out]
    }
    frame Error {
      n173 = local write "error out"(w285) -> ()
    }
  }
  n174 = xnode "Read/Write Control"("FPGA VI Reference In"=w23, "PFI2"=w14, "PFI3"=w14) -> ("FPGA VI Reference Out"=w13:refnum<k20>)  [unwired: 1 in, 1 out]
  n175 = xnode "Close FPGA VI Reference"("FPGA VI Reference In"=w13) -> ()  [unwired: 1 in, 1 out]
